vi "Interface_Asset_Read Process Name.vi"(11 "Load in":refnum<class "Load.lvclass">) -> (2 "Process Name":string, 3 "Load out":refnum<class "Load.lvclass">)   [LabVIEW 2015, in "Load.lvclass"]
uses:
  Load.lvclass
  Load.lvclass/Load.ctl
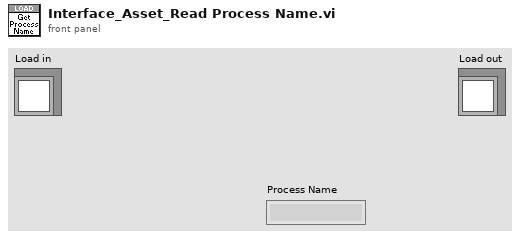
[diagram p1: front panel]
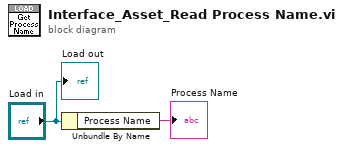
[diagram p0: block diagram]
diagram:
  n1 = Unbundle By Name("Load in") -> ("Process Name"=→"Process Name":string)
  "Load out" <- "Load in"
